vi "joystick to degree.vi"(9 "x":dbl, 11 "y":dbl) -> (3 "Degree":dbl)   [LabVIEW 2014]
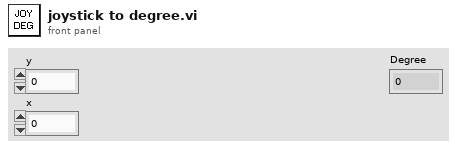
[diagram p1: front panel]
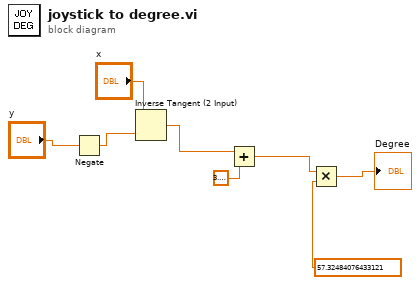
[diagram p0: block diagram]
diagram:
  n1 = Negate(x="y") -> (-x=w1:dbl)
  n2 = Inverse Tangent (2 Input)(1:w1, 2:"x") -> (0:w4:dbl)
  n3 = Add(x=w4, y=3.141592653589793) -> (x+y=w3:dbl)
  n4 = Multiply(x=w3, y=57.32484076433121) -> (x*y=→"Degree":dbl)
